vi "calcHorizontalRadius.vi"(1 "Y Coordinate":i32=238, 2 "X Coordinate":i32=322, 3 "Vertical radius":i32=322, 4 "Source Image":T1(plugin-control)) -> (0 "mean radius":dbl)   [LabVIEW 2009, in "ImageAnalysis.lvlib"]
uses:
  ImageAnalysis.lvlib
  <vilib>/vision/NI_Vision_Development_Module.lvlib
panel:
  out "radius(pos)":i32
  out "Pixel Value (U8) 2":u8
  out "radius(neg)":i32
  out "Pixel Value (U8)":u8
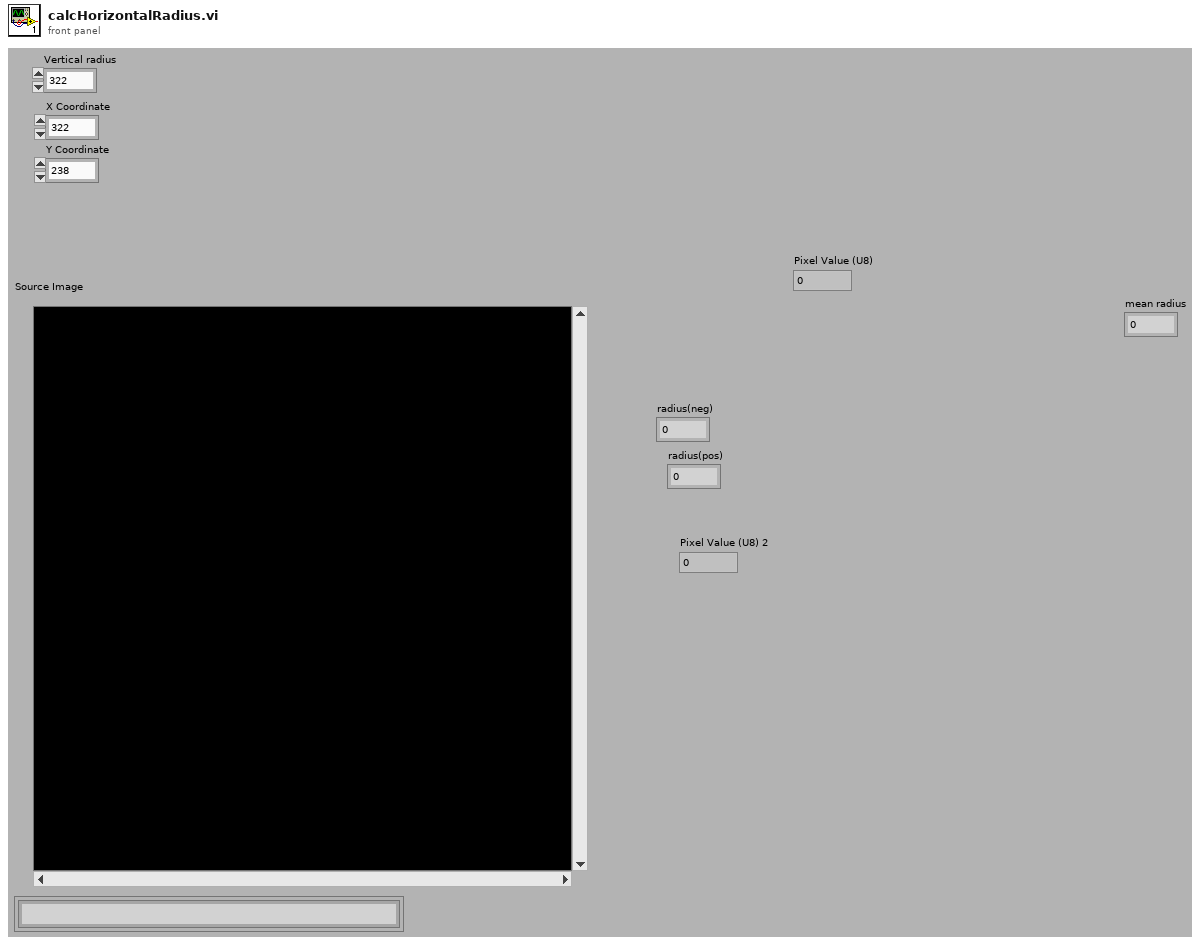
[diagram p1: front panel]
types:
  T1 = typedef "IMAQ Image.ctl" = refnum<image>
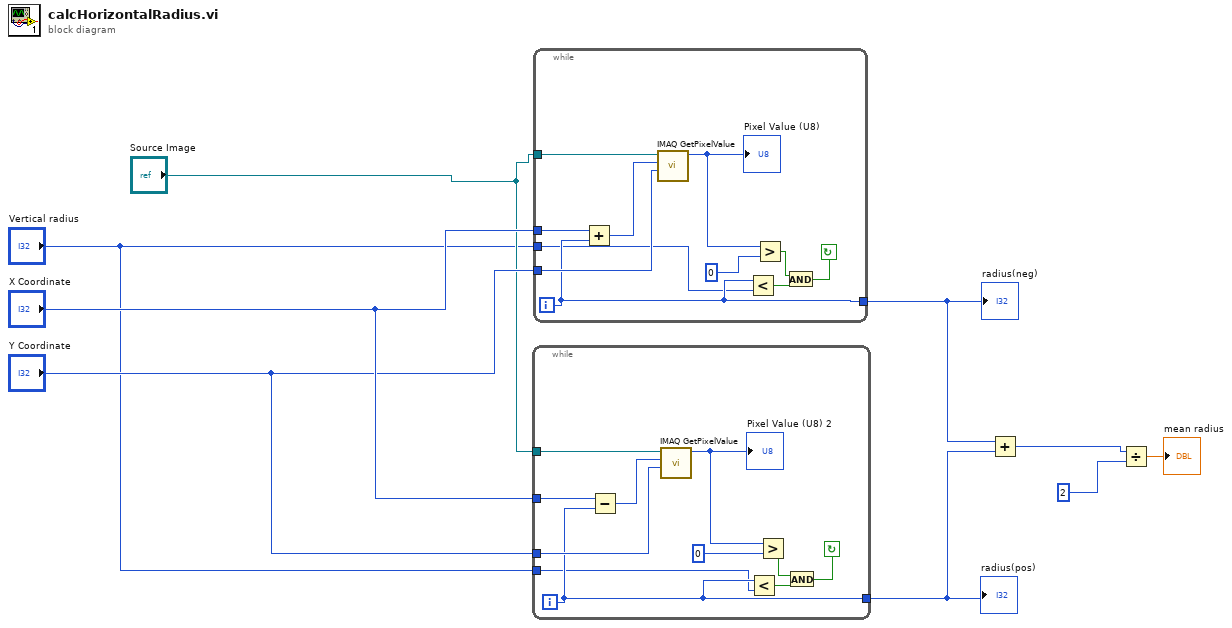
[diagram p0: block diagram]
diagram:
  n1 = while {
    tunnel: "Source Image" -> [w20]
    tunnel: [w11] -> w9
    tunnel: "X Coordinate" -> [w16]
    tunnel: "Y Coordinate" -> [w15]
    tunnel: "Vertical radius" -> [w10]
    i -> [w11]
    stop <- w13 continue-if-true
    n2 = Subtract(x=w16, y=w11) -> (x-y=w17:i32)
    n3 = call "IMAQ GetPixelValue"("Image"=w20, "X Coordinate"=w17, "Y Coordinate"=w15) -> ("Pixel Value (U8)"=w19:u8)  [unwired: 3 in, 4 out]
    "Pixel Value (U8) 2" <- w19
    n4 = Less?(x=w11, y=w10) -> (x < y?=w12:bool)
    n5 = Greater?(x=w19, y=u8 0) -> (0:w14:bool)
    n6 = And(x=w14, y=w12) -> (x .and. y?=w13:bool)
  }
  "radius(pos)" <- w9
  n7 = while {
    tunnel: "Source Image" -> [w31]
    tunnel: [w22] -> w8
    tunnel: "X Coordinate" -> [w28]
    tunnel: "Y Coordinate" -> [w26]
    tunnel: "Vertical radius" -> [w21]
    i -> [w22]
    stop <- w24 continue-if-true
    n8 = Add(x=w28, y=w22) -> (x+y=w27:i32)
    n9 = call "IMAQ GetPixelValue"("Image"=w31, "X Coordinate"=w27, "Y Coordinate"=w26) -> ("Pixel Value (U8)"=w30:u8)  [unwired: 3 in, 4 out]
    "Pixel Value (U8)" <- w30
    n10 = Less?(x=w22, y=w21) -> (x < y?=w23:bool)
    n11 = Greater?(x=w30, y=u8 0) -> (0:w25:bool)
    n12 = And(x=w25, y=w23) -> (x .and. y?=w24:bool)
  }
  "radius(neg)" <- w8
  n13 = Add(x=w8, y=w9) -> (x+y=w7:i32)
  n14 = Divide(x=w7, y=2) -> (x/y=→"mean radius":dbl)
